vi "rvc blending function.vi"(9 "Numeric 5":dbl, 10 "Numeric 6":dbl, 11 "Numeric 4":dbl) -> (1 "Numeric":dbl, 2 "Numeric 2":dbl, 3 "Numeric 3":dbl)   [LabVIEW 2013]
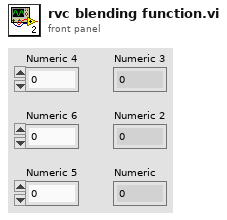
[diagram p1: front panel]
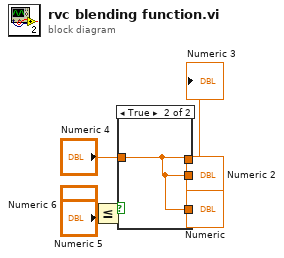
[diagram p0: block diagram]
diagram:
  n1 = Less Or Equal?(x="Numeric 6", y="Numeric 5") -> (x <= y?=w2:bool)
  n2 = case shown="True" w2 {
    tunnel: [_ w8] -> w5
    tunnel: "Numeric 4" -> [_ w8]
    tunnel: [_ w8] -> w6
    tunnel: [_ w8] -> w7
    frame False {
    }
    frame True {
    }
  }
  "Numeric" <- w7
  "Numeric 2" <- w6
  "Numeric 3" <- w5
